vi "Measure.vi"(0 "AbstractDMM in":refnum<class "Abstract_Instrument.lvclass">, 5 "Measure_Parameters":variant, 11 "error in (no error)":errorcluster) -> (4 "AbstractDMM out":refnum<class "Abstract_Instrument.lvclass">, 6 "Measure_Results":variant, 15 "error out":errorcluster)   [LabVIEW 2020, in "Abstract_Instrument.lvlib" / "Abstract_Instrument.lvclass"]
uses:
  Abstract_Instrument.lvclass
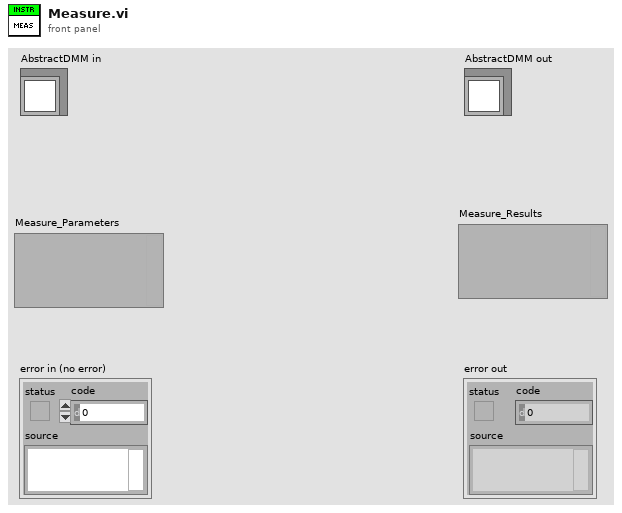
[diagram p1: front panel]
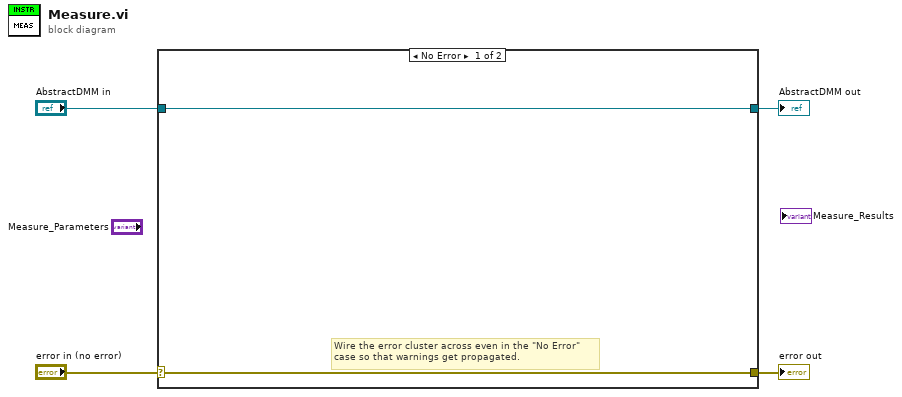
[diagram p0: block diagram]
diagram:
  n1 = case shown="No Error" "error in (no error)" {
    selector: "error in (no error)" -> [w5 w8]
    tunnel: [w5 w8] -> w3
    tunnel: [w6 w7] -> w1
    tunnel: "AbstractDMM in" -> [w6 w7]
    frame No Error {
      # "Wire the error cluster across even in the \"No Error\"\ncase so that warnings get propagated."
    }
    frame Error {
    }
  }
  "error out" <- w3
  "AbstractDMM out" <- w1
